vi "Load Config.vi"(8 "error in (no error)":errorcluster, 11 "VoltageOutChannel in":refnum<class "VoltageOutChannel.lvclass">) -> (0 "error out":errorcluster, 3 "VoltageOutChannel out":refnum<class "VoltageOutChannel.lvclass">)   [LabVIEW 2020, in "VolatusDAQConfig.lvlib" / "VoltageOutChannel.lvclass"]
uses:
  VoltageOutChannel.lvclass
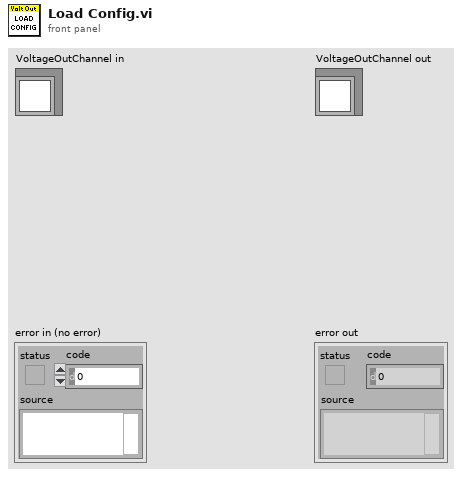
[diagram p1: front panel]
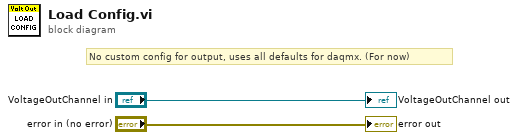
[diagram p0: block diagram]
diagram:
  # "No custom config for output, uses all defaults for daqmx. (For now)"
  "error out" <- "error in (no error)"
  "VoltageOutChannel out" <- "VoltageOutChannel in"
